vi "Assign Insertion Ramping v2.vi"(0 "Ramp Time [sec]":dbl=3.0, 1 "end":dbl=1.0 format="%0.2f", 2 "start":dbl format="%0.2f", 3 "Target Tool Insertion Speed":dbl=1.0, 4 "Robot In":i32) -> (8 "actInsertionLength":dbl)   [LabVIEW 2016]
uses:
  <vilib>/Analysis/1siggen.llb/Ramp Pattern by Samples.vi
  Subsystems/Global Variables.vi
  <vilib>/Analysis/NI_AALBase.lvlib
panel:
  out "32bit integer":i32
  out "Numeric":i32
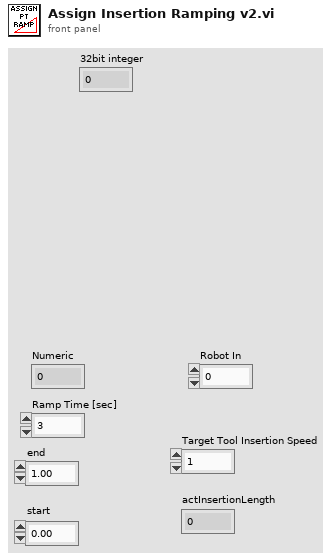
[diagram p1: front panel]
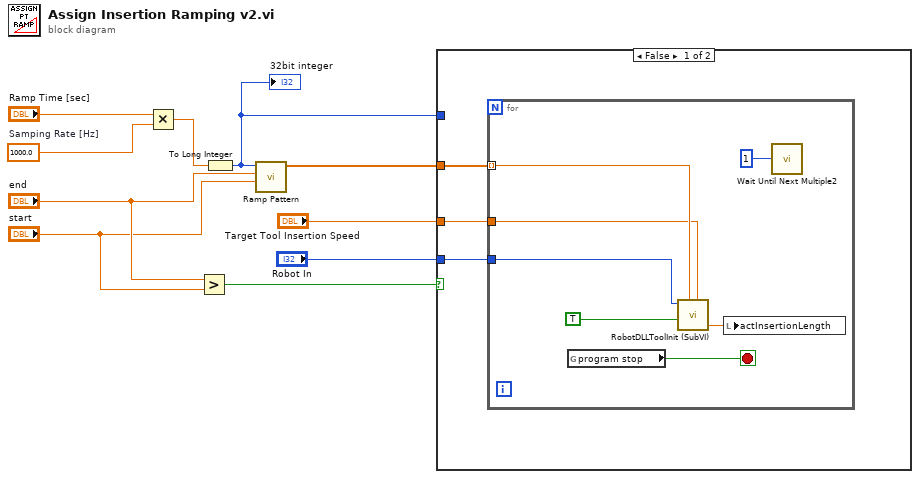
[diagram p0: block diagram]
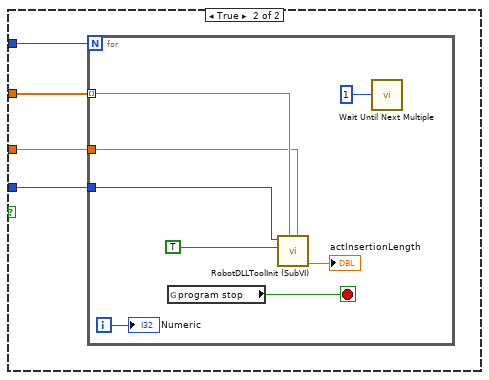
[diagram p2: hidden frame]
diagram:
  w9 = 1000.0  # Samping Rate [Hz]
  n1 = Multiply(x="Ramp Time [sec]", y=w9) -> (x*y=w8:dbl)
  n2 = Greater?(x="end", y="start") -> (0:w5:bool)
  n3 = To Long Integer(number=w8) -> (32bit integer=w7:i32)
  "32bit integer" <- w7
  n4 = call-poly <vilib>:"Ramp Pattern.vi"("start"="start", "end"="end", "samples"=w7) -> ("Ramp Pattern"=w6:dbl[])  [unwired: 7 in, 1 out]
  n5 = case shown="False" w5 {
    tunnel: w7 -> [_ w24]
    tunnel: w6 -> [w12 w23]
    tunnel: "Robot In" -> [w13 w22]
    tunnel: "Target Tool Insertion Speed" -> [w11 w21]
    frame False {
      n6 = for {
        tunnel: w13 -> [w17]
        tunnel: w12 -> [w16] mode=indexing
        tunnel: w11 -> [w15]
        stop <- w19 stop-if-true
        n7 = global read "Global Variables.vi" "program stop"() -> (w19:bool)
        n8 = call "RobotDLLToolInit (SubVI).vi"("Target Tool Insertion Speed"=w15, "Target Tool Insertion Length"=w16, "Tool Withdraw"=TRUE ("Tool Insertion"), "ArmID"=w17) -> ("actInsertionLength"=w14:dbl)  [unwired: 7 in]
        n9 = local write "actInsertionLength"(w14) -> ()
        n10 = call "Wait Until Next Multiple2"("Count(mSec)"=u32 1) -> ()  [unwired: 1 out]
      }
    }
    frame True {
      n11 = for {
        N: w24 -> [_]
        tunnel: w23 -> [w31] mode=indexing
        tunnel: w22 -> [w26]
        tunnel: w21 -> [w25]
        i -> [w27]
        stop <- w28 stop-if-true
        n12 = global read "Global Variables.vi" "program stop"() -> (w28:bool)
        n13 = call "RobotDLLToolInit (SubVI).vi"("Target Tool Insertion Speed"=w25, "Target Tool Insertion Length"=w31, "Tool Insertion"=TRUE, "ArmID"=w26) -> ("actInsertionLength"=→"actInsertionLength":dbl)  [unwired: 7 in]
        n14 = call "Wait Until Next Multiple"("Count(mSec)"=u32 1) -> ()  [unwired: 1 out]
        "Numeric" <- w27
      }
    }
  }
